vi "mmWave Adapter 2 to Adapter Chain.vi"(7 "mmWave Adapters":T1[](array[typedef])) -> (8 "Adapter Chain Array":T2[](array[typedef]))   [LabVIEW 2019]
uses:
  <instrlib>/niMmWave/ni3620/Config/v1/Host/Public/Typedefs/mmWave Adapter Chain.ctl
  <instrlib>/niMmWave/ni3620/Config/v1/Host/Public/Typedefs/mmWave Adapter 2.ctl
  <instrlib>/niMmWave/ni3620/Config/v1/Host/niMmWave Config v1 Host.lvlib
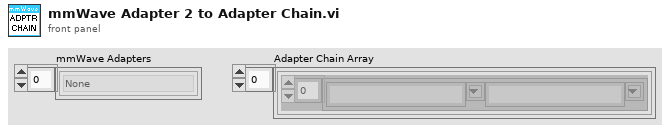
[diagram p1: front panel]
types:
  T1 = typedef "niMmWave Config v1 Host.lvlib/mmWave Adapter 2.ctl" = enum16{"None", "NI 3647 71-76 GHz", "NI 3657 71-76 GHz", "NI 5580 55-68 GHz", "NI 5580 55-68 GHz Prototype Deck", "NI 3602 27.5-29.5 GHz", "NI 3642 27.5-29.5 GHz", "NI 3652 27.5-29.5 GHz", "NI 3603 37.0-43.5 GHz", "NI 3643 37.0-43.5 GHz", "NI 3653 37.0-43.5 GHz", "NI 3602 24.25-33.40 GHz", "NI 3642 24.25-33.40 GHz", "NI 3652 24.25-33.40 GHz"}
  T2 = typedef "niMmWave Config v1 Host.lvlib/mmWave Adapter Chain.ctl" = cluster{"mmWave adapters":string[]}
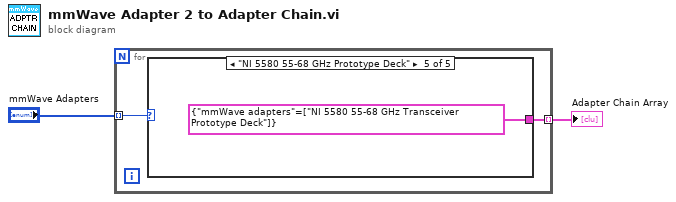
[diagram p0: block diagram]
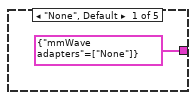
[diagram p2: hidden frame]
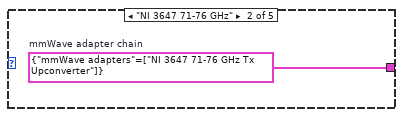
[diagram p3: hidden frame]
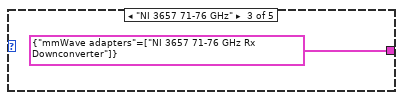
[diagram p4: hidden frame]
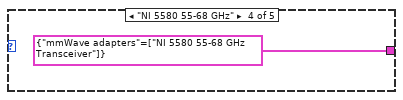
[diagram p5: hidden frame]
diagram:
  n1 = for {
    tunnel: "mmWave Adapters" -> [w4] mode=indexing
    tunnel: [w3] -> w2 mode=indexing
    n2 = case shown="\"NI 5580 55-68 GHz Prototype Deck\"" w4 {
      tunnel: [T2 {"mmWave adapters"=["None"]} ("mmWave adapter chain") w6 T2 {"mmWave adapters"=["NI 3657 71-76 GHz Rx Downconverter"]} ("mmWave adapter chain") T2 {"mmWave adapters"=["NI 5580 55-68 GHz Transceiver"]} ("mmWave adapter chain") T2 {"mmWave adapters"=["NI 5580 55-68 GHz Transceiver Prototype Deck"]} ("mmWave adapter chain")] -> w3
      frame "None", Default {
      }
      frame "NI 3647 71-76 GHz" {
        w6 = T2 {"mmWave adapters"=["NI 3647 71-76 GHz Tx Upconverter"]}  # mmWave adapter chain
      }
      frame "NI 3657 71-76 GHz" {
      }
      frame "NI 5580 55-68 GHz" {
      }
      frame "NI 5580 55-68 GHz Prototype Deck" {
      }
    }
  }
  "Adapter Chain Array" <- w2
